vi "SENS_IF_GAIN_STAT.vi"(0 "VISA IN":refnum<visa-resource-name>, 1 "ID":string, 5 "error in":errorcluster, 7 "Channel":i32) -> (14 "VISA Out":refnum<visa-resource-name>, 16 "Data":string, 19 "error out":errorcluster)   [LabVIEW 2018, in "PNA-X.lvlib"]
doc: "SENSe<cnum>:IF:GAIN[:STATe]?, <id> \n(Read only) Returns the gain state for the specified receiver. Use SENS:IF:GAIN:ALL. to set the gain \nstate for all channels. \nParameters \n<cnum> Existing channel number to manipulate. If unspecified, <cnum> is set to 1. \n<id> Choose from: 'A', 'B', 'R1', 'R2'. \nNote: The A and R1 receivers are always switched together. B and R2 are also \nalways switched together. For example, if you specify 'A', R1 will also be \nswitched. \nExamples SENS:IF:GAIN? 'A' \nReturn Type Boolean \nDefault Not Applicable \n1751"
uses:
  PNA-X.lvlib
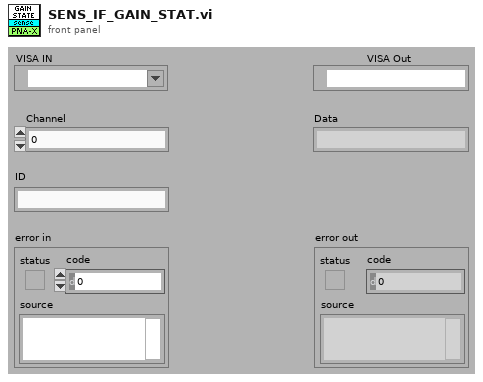
[diagram p1: front panel]
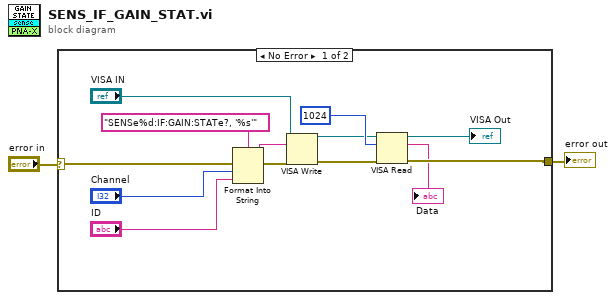
[diagram p0: block diagram]
diagram:
  n1 = case shown="No Error" "error in" {
    selector: "error in" -> [w15 w16]
    tunnel: [w6 w16] -> w1
    frame No Error {
      n2 = Format Into String(format string="SENSe%d:IF:GAIN:STATe?, '%s'" ("Cmdline"), error in=w15, "Channel", "ID") -> (resulting string=w13:string, error out=w14:errorcluster)  [unwired: 1 in]
      n3 = VISA Write(VISA resource name="VISA IN", write buffer=w13, error in (no error)=w14) -> (VISA resource name out=w8:refnum<visa-resource-name>, error out=w10:errorcluster)  [unwired: 1 out]
      n4 = VISA Read(VISA resource name=w8, byte count=1024, error in (no error)=w10) -> (VISA resource name out=→"VISA Out":refnum<visa-resource-name>, read buffer=→"Data":string, error out=w6:errorcluster)  [unwired: 1 out]
    }
    frame Error {
    }
  }
  "error out" <- w1
